vi "Launch Client Loop.vi"(8 "error in (no error)":errorcluster, 11 "VISA Client in":refnum<class "Serial Client.lvclass">) -> (0 "error out":errorcluster, 3 "VISA Client out":refnum<class "Serial Client.lvclass">)   [LabVIEW 2020, in "Stream-Serial.lvlib" / "Serial Client.lvclass"]
uses:
  Serial Client.lvclass
  Client Loop Async.vi
  lv-stream/stream/Connection/Connection.lvclass
  lv-stream/stream/Connection/State.ctl
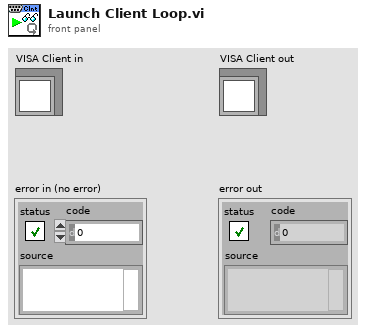
[diagram p1: front panel]
types:
  T1 = typedef "Stream.lvlib/Connection.lvclass/State.ctl" = enum16{"Closed", "Idle", "Connecting", "Connected", "Shutdown"}
  T2 = typedef "Stream-Serial.lvlib/Serial Client.lvclass/Ref Data.ctl" = cluster{"Stream":refnum<class "Serial Stream.lvclass">, "Client Loop":refnum<vi>, "Port Config":T3, "VISA Resource":refnum<visa-resource-name>}
  T3 = typedef "Stream-Serial.lvlib/Serial Client.lvclass/Port Config.ctl" = cluster{"Baud (115200)":u32, "Data Bits (8)":u8, "Stop Bits (1)":T4, "Flow Control":T5, "Use LineTerm?":bool, "LineTerm (\\n)":string, "Timeout ms (10000)":i32, "Parity (None)":T6}
  T4 = typedef "Stream-Serial.lvlib/Serial Client.lvclass/Stop Bits.ctl" = u16
  T5 = typedef "Stream-Serial.lvlib/Serial Client.lvclass/Flow Control.ctl" = u16
  T6 = typedef "Stream-Serial.lvlib/Serial Client.lvclass/Parity.ctl" = enum16{"None", "Odd", "Even", "Mark", "Space"}
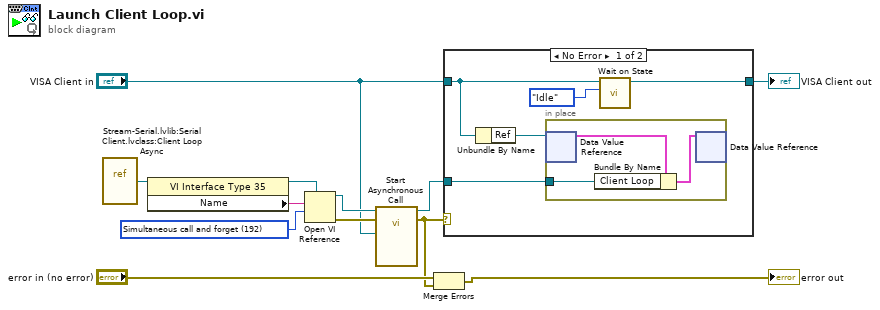
[diagram p0: block diagram]
diagram:
  w9 = 192 items=["Record modifications"=1, "Open templates for editing"=2, "Prompt user to save"=4, "Prepare for reentrant run"=8, "Prompt to find missing subVIs"=16, "Hide loading dialog box"=32, "Enable simultaneous calls"=64, "Prepare to call and forget"=128, "Simultaneous call and forget"=192, "Prepare to call and collect"=256, "Simultaneous call and collect"=320]
  n1 = vi-ref "Stream-Serial.lvlib:Serial Client.lvclass:Client Loop Async.vi"() -> (w7:refnum<vi>)
  n2 = property class="VI Interface Type 35"(reference=w7) -> (reference out=w10:refnum<vi>, "Name"=w8:string)  [unwired: 1 in, 1 out]
  n3 = Open VI Reference(type specifier VI Refnum (for type only)=w10, vi path=w8, options=w9) -> (vi reference=w12:refnum<vi>, error out=w11:errorcluster)  [unwired: 3 in]
  n4 = call-by-ref "Start Asynchronous Call"(reference=w12, error in=w11, "VISA Client in"="VISA Client in") -> (reference out=w4:refnum<vi>, error out=w3:errorcluster)  [unwired: 11 in]
  n5 = Merge Errors("error in (no error)", w3) -> (→"error out":errorcluster)
  n6 = case shown="No Error" w3 {
    tunnel: w4 -> [w16 _]
    tunnel: "VISA Client in" -> [w14 w21]
    tunnel: [w15 w21] -> w1
    frame No Error {
      n7 = Unbundle By Name(w14) -> ("Ref"=w17:refnum<data-value>)
      n8 = in-place {
        in-place-border: w16 -> [w18]
        n9 = in-place-dvr #1(w17) -> (w20:T2)  [unwired: 1 out]
        n10 = Bundle By Name(cluster=w20, "Client Loop"=w18) -> (w19:T2)
        n11 = in-place-dvr #1(w19) -> ()  [unwired: 2 out]
      }
      n12 = call "Wait on State.vi"("State"=State."Idle", "Connection in"=w14) -> ("Connection out"=w15:refnum<class "Serial Client.lvclass">)  [unwired: 7 in, 2 out]
    }
    frame Error {
    }
  }
  "VISA Client out" <- w1
